vi "Bury - Simple.vi"() -> ()   [LabVIEW 2017]
doc: "A demonstration of burying the Corpse (legacy) at the grave (Diagram Disable Structure). This includes step-by-step instructions for removing the grave and leaving only the Spirit (refactored) code behind with one of two methods: shortcut menu plugin or Quick Drop shortcut plugin."
panel:
  out "Any?":bool
  in  "Input":bool[](array[boolean])=[FALSE, FALSE, FALSE, FALSE, TRUE, FALSE, FALSE]
  # "Overview: Demonstrates burying the legacy code\nInstructions:\n1. Run the VI\n2. Observe the value of the Any? indicator\n3. Uncheck the TRUE element in the Input array\n4. Run the VI\n5. Observe the value of the Any? indicator\n6. Switch to the block diagram and follow the instructions to remove the legacy code"
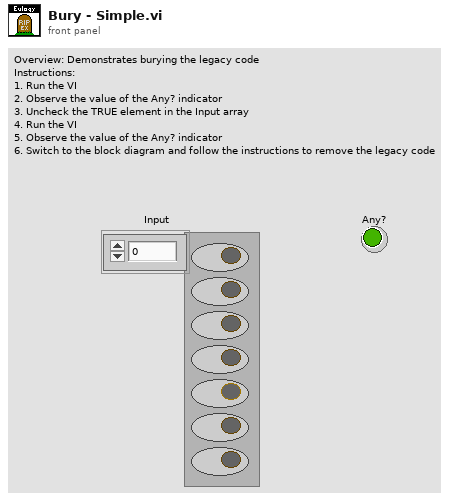
[diagram p1: front panel]
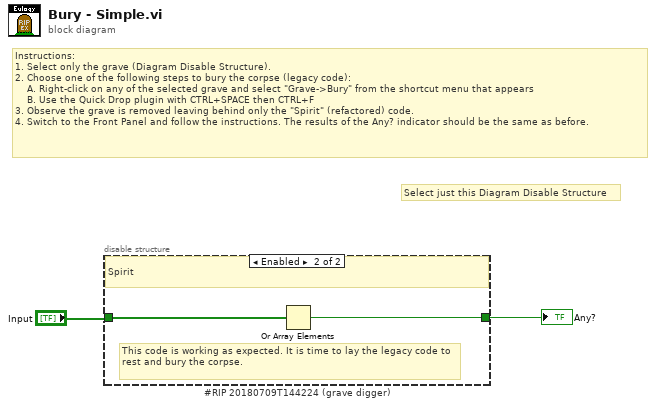
[diagram p0: block diagram]
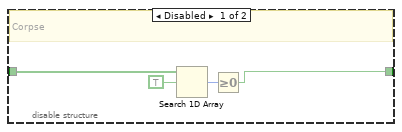
[diagram p2: hidden frame]
diagram:
  # "Select just this Diagram Disable Structure"
  # "Instructions:\n1. Select only the grave (Diagram Disable Structure).\n2. Choose one of the following steps to bury the corpse (legacy code):\n    A. Right-click on any of the selected grave and select \"Grave->Bury\" from the shortcut menu that appears\n    B. Use the Quick Drop plugin with CTRL+SPACE then CTRL+F\n3. Observe the grave is removed leaving behind only the \"Spirit\" (refactored) code.\n4. Switch to the Front Panel and follow the instructions. The results of the Any? indicator should be the same as before."
  n1 = disable-structure "#RIP 20180709T144224 (grave digger)" shown="Enabled" {
    disable-tunnel: "Input" -> [w6 w8]
    disable-tunnel: [w5 w7] -> w1
    frame Disabled {
      # "Corpse"
      n2 = Search 1D Array(1D array=w6, element=TRUE) -> (index of element=w3:i32)  [unwired: 1 in]
      n3 = Greater Or Equal To 0?(x=w3) -> (x >= 0?=w5:bool)
    }
    frame Enabled {
      # "This code is working as expected. It is time to lay the legacy code to rest and bury the corpse."
      # "Spirit"
      n4 = Or Array Elements(Boolean array=w8) -> (logical OR=w7:bool)
    }
  }
  "Any?" <- w1
